vi "WSVCAP SHL Host LL RFFE Build and Parse Data.vi"(0 "Data Out":string, 1 "Data Out (Cycle Commands)":string[](array[string]), 2 "Post Command Delay":dbl[](array[numeric]) format="%#.0p s", 5 "Data Out (Unique)":string[](array[string]), 9 "RFFE Data In [U8]":u8[][](array[numeric]) format="%02x", 12 "Simulate FPGA (Cycle Only)":bool, 13 "DUT Mask (All)":bool[](array[boolean])=[TRUE, TRUE, TRUE, TRUE, TRUE, TRUE, TRUE, TRUE, TRUE, TRUE, TRUE, TRUE, TRUE, TRUE, TRUE, TRUE]) -> (4 "RFFE Data Out [U8]":u8[][](array[numeric]) format="%02x", 6 "CMD Lengths (Bits)":u8[](array[numeric]), 8 "CMD Delays (Ticks)":u32[](array[numeric]), 10 "RFFE Data In":string[](array[string]))   [LabVIEW 2012]
panel:
  # "DUT 01"
  # "DUT 02"
  # "DUT 03"
  # "DUT 04"
  # "DUT 05"
  # "DUT 06"
  # "DUT 07"
  # "DUT 08"
  # "DUT 09"
  # "DUT 10"
  # "DUT 11"
  # "DUT 12"
  # "DUT 13"
  # "DUT 14"
  # "DUT 15"
  # "DUT 16"
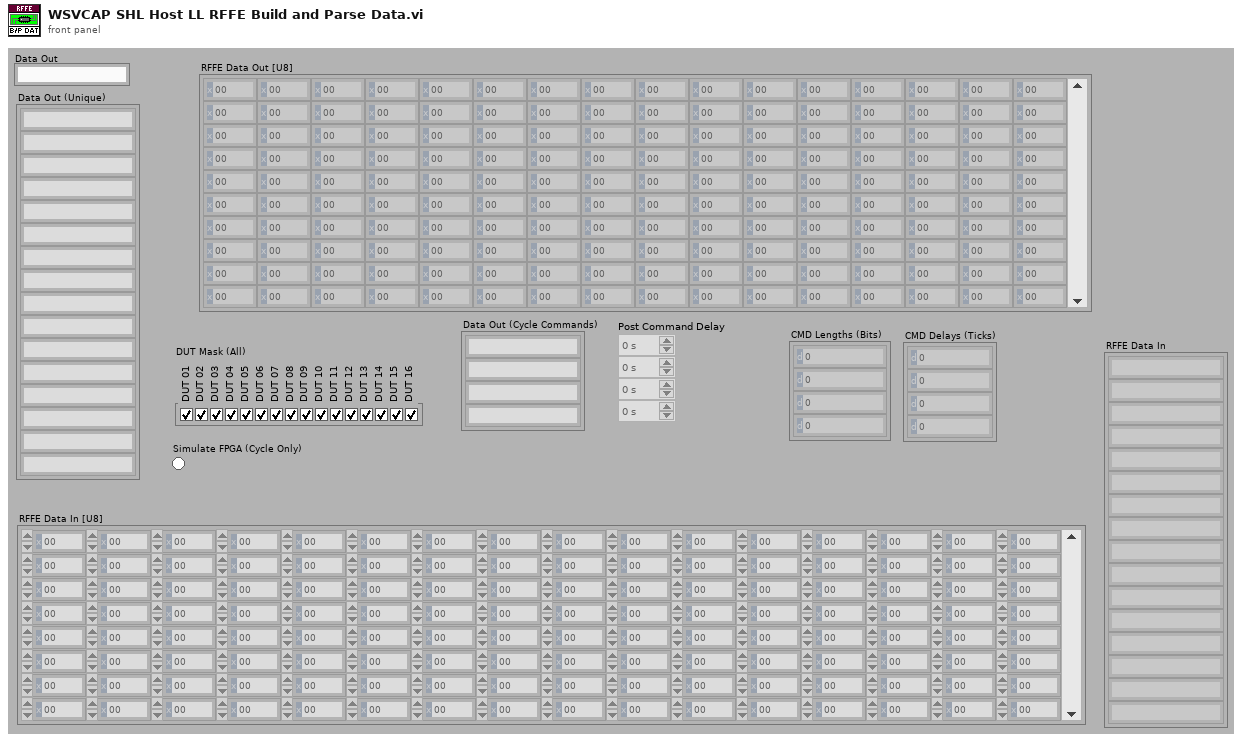
[diagram p1: front panel]
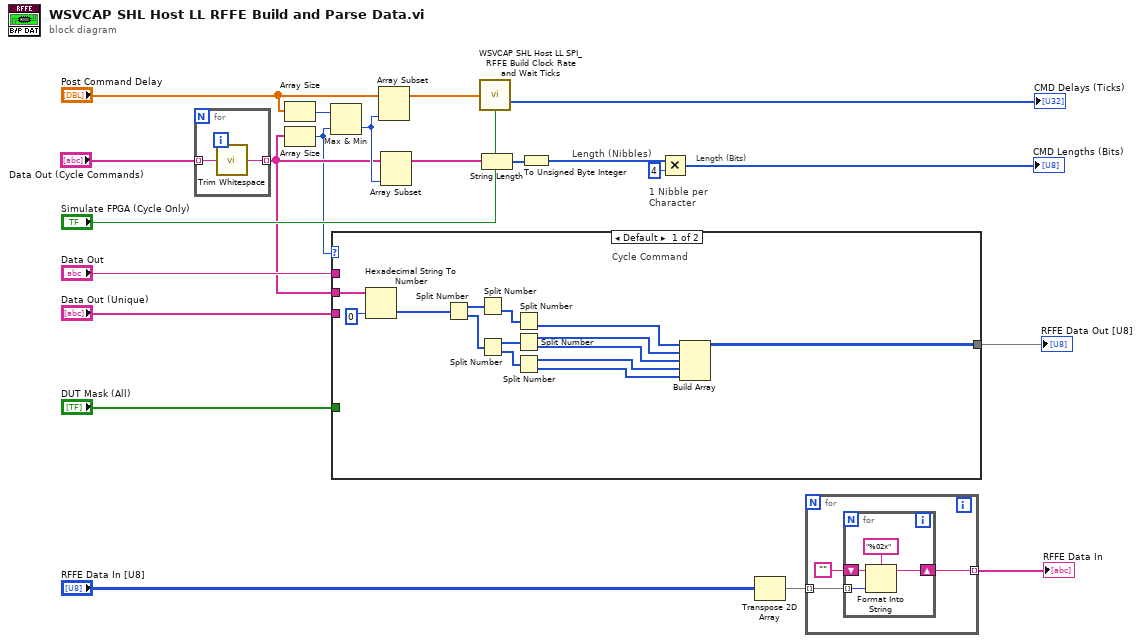
[diagram p0: block diagram]
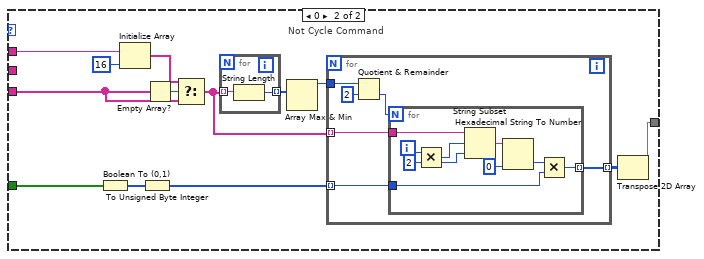
[diagram p2: hidden frame]
diagram:
  # "Length (Bits)"
  # "Length (Nibbles)"
  # "1 Nibble per Character"
  n1 = for {
    tunnel: "Data Out (Cycle Commands)" -> [w23] mode=indexing
    tunnel: [w22] -> w2 mode=indexing
    n2 = call <vilib>:"Trim Whitespace.vi"("string"=w23) -> ("trimmed string"=w22:string)  [unwired: 1 in]
  }
  n3 = Array Size(array="Post Command Delay") -> (size(s)=w12:i32)
  n4 = Array Size(array=w2) -> (size(s)=w1:i32)
  n5 = Max & Min(x=w12, y=w1) -> (min(x,y)=w9:i32)  [unwired: 1 out]
  n6 = case shown="Default" w1 {
    tunnel: "DUT Mask (All)" -> [_ w50]
    tunnel: "Data Out (Unique)" -> [_ w43]
    tunnel: [w29 w42] -> w17
    tunnel: "Data Out" -> [_ w38]
    tunnel: w2 -> [w37 _]
    frame Default {
      # "Cycle Command"
      n7 = Hexadecimal String To Number(string=w37, default (0uL)=u64 0 ("Read Data")) -> (number=w30:u64[])  [unwired: 1 in, 1 out]
      n8 = Split Number(x=w30) -> (hi(x)=w35:u32[], lo(x)=w34:u32[])
      n9 = Split Number(x=w35) -> (lo(x)=w33:u16[])  [unwired: 1 out]
      n10 = Split Number(x=w34) -> (hi(x)=w32:u16[], lo(x)=w31:u16[])
      n11 = Split Number(x=w33) -> (lo(x)=w28:u8[])  [unwired: 1 out]
      n12 = Split Number(x=w32) -> (hi(x)=w27:u8[], lo(x)=w26:u8[])
      n13 = Split Number(x=w31) -> (hi(x)=w25:u8[], lo(x)=w24:u8[])
      n14 = Build Array(w28, w27, w26, w25, w24) -> (w29:u8[][])
    }
    frame 0 {
      # "Not Cycle Command"
      n15 = Boolean To (0,1)(Boolean=w50) -> (0, 1=w49:i16[])
      n16 = Initialize Array(w38, 16 ("dimension size")) -> (w44:string[])
      n17 = To Unsigned Byte Integer(number=w49) -> (unsigned 8bit integer=w48:u8[])
      n18 = Empty Array?(array=w43) -> (empty?=w46:bool)
      n19 = Select(t=w44, s=w46, f=w43) -> (s? t:f=w41:string[])
      n20 = for {
        tunnel: w41 -> [w52] mode=indexing
        tunnel: [w51] -> w40 mode=indexing
        n21 = String Length(string=w52) -> (length=w51:i32)
      }
      n22 = Array Max & Min(array=w40) -> (max value=w39:i32)  [unwired: 3 out]
      n23 = for {
        tunnel: w48 -> [w56] mode=indexing
        tunnel: [w55] -> w47 mode=indexing
        tunnel: w41 -> [w54] mode=indexing
        tunnel: w39 -> [w53]
        n24 = Quotient & Remainder(x=w53, y=2) -> (floor(x/y)=w57:i32)  [unwired: 1 out]
        n25 = for {
          N: w57 -> [_]
          tunnel: w54 -> [w67]
          tunnel: [w60] -> w55 mode=indexing
          tunnel: w56 -> [w61]
          i -> [w66]
          w64 = 2 ("y")
          n26 = Multiply(x=w66, y=w64) -> (x*y=w65:i32)
          n27 = String Subset(string=w67, offset (0)=w65, length (rest)=w64) -> (substring=w63:string)
          n28 = Hexadecimal String To Number(string=w63, default (0uL)=u8 0 ("default (0 U32)")) -> (number=w59:u8)  [unwired: 1 in, 1 out]
          n29 = Multiply(x=w59, y=w61) -> (x*y=w60:u8)
        }
      }
      n30 = Transpose 2D Array(2D array=w47) -> (transposed array=w42:u8[][])
    }
  }
  "RFFE Data Out [U8]" <- w17
  n31 = Array Subset(array="Post Command Delay", length=w9) -> (w10:dbl[])  [unwired: 1 in]
  n32 = Array Subset(array=w2, length=w9) -> (w8:string[])  [unwired: 1 in]
  n33 = call "WSVCAP SHL Host LL SPI_RFFE Build Clock Rate and Wait Ticks.vi"("CMD Delay (s)"=w10, "Simulate FPGA"="Simulate FPGA (Cycle Only)") -> ("CMD Delay (Ticks)"=→"CMD Delays (Ticks)":u32[])  [unwired: 10 in, 3 out]
  n34 = String Length(string=w8) -> (length=w16:i32[])
  n35 = To Unsigned Byte Integer(number=w16) -> (unsigned 8bit integer=w13:u8[])
  n36 = Multiply(x=w13, y=u8 4 ("Read Data")) -> (x*y=→"CMD Lengths (Bits)":u8[])
  n37 = Transpose 2D Array(2D array="RFFE Data In [U8]") -> (transposed array=w20:u8[][])
  n38 = for {
    tunnel: w20 -> [w70] mode=indexing
    tunnel: [w68] -> w19 mode=indexing
    n39 = for {
      tunnel: w70 -> [w74] mode=indexing
      shift-right: [w72] -> w68
      shift-left: "" -> [w71]
      n40 = Format Into String(format string="%02x", initial string=w71, w74) -> (resulting string=w72:string)  [unwired: 1 in, 1 out]
    }
  }
  "RFFE Data In" <- w19
